vi "DIAdem Enqueue Request.vi"(7 "Queue Entry":enum16{"Front", "Back"}(ring), 8 "error in (no error)":errorcluster, 9 "timeout in ms (300000)":i32=300000, 10 "Wait for Completion? (f)":bool, 11 "DD_Report":T1) -> (0 "error out":errorcluster, 2 "timed out?":bool, 3 "Results":string)   [LabVIEW 2011]
uses:
  DIAdem Daemon Queue.ctl
  DIAdem Daemon Script Type.ctl
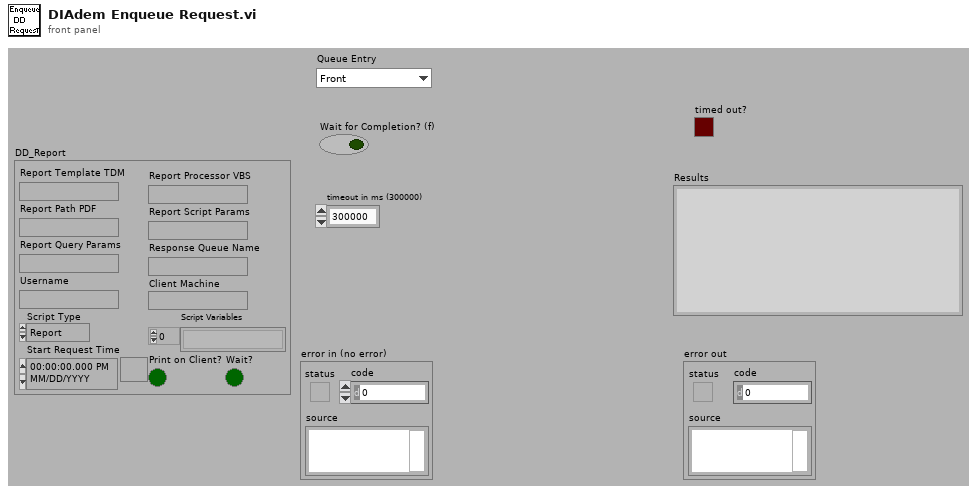
[diagram p1: front panel]
types:
  T1 = typedef "DIAdem Daemon Queue.ctl" = cluster{"Report Template TDM":path, "Report Processor VBS":path, "Report Path PDF":path, "Report Script Params":string, "Username":string, "Script Type":T2, "Report Query Params":string, "Client Machine":string, "Print on Client?":bool, "Response Queue Name":string, "Script Variables":string[], "Start Request Time":timestamp, "Wait?":bool}
  T2 = typedef "DIAdem Daemon Script Type.ctl" = enum16{"Report", "Query", "Script", "Datasheet", "Append", "Restart", "Stop"}
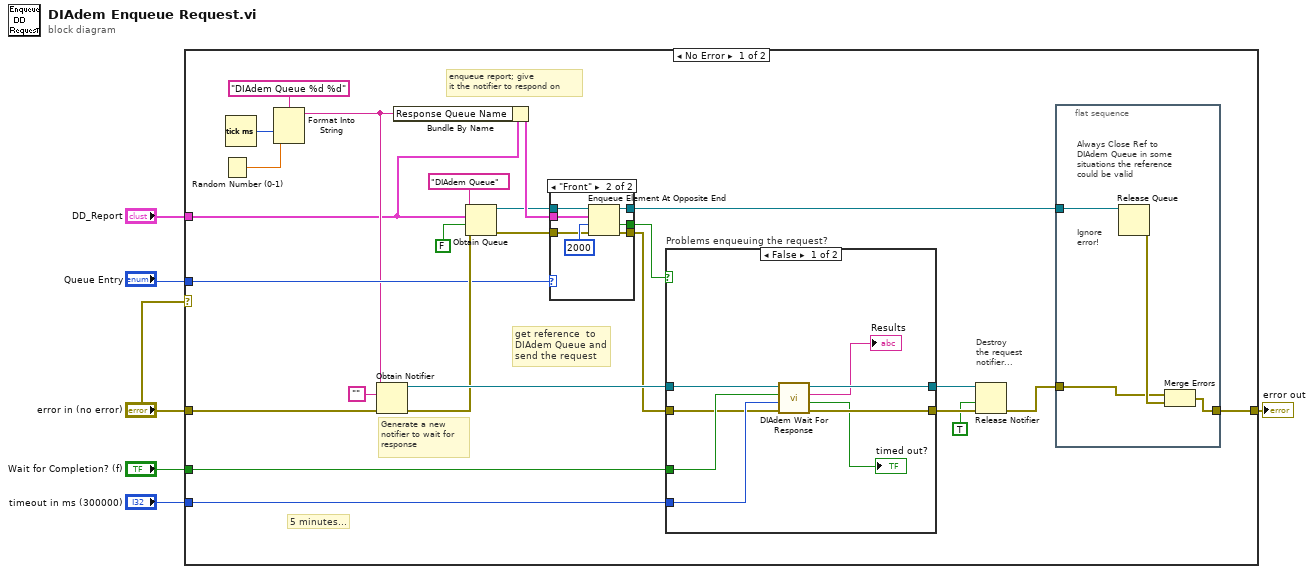
[diagram p0: block diagram]
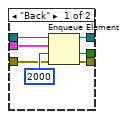
[diagram p2: hidden frame]
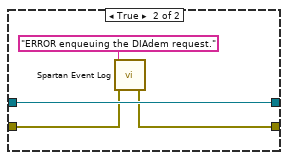
[diagram p3: hidden frame]
diagram:
  n1 = case shown="No Error" "error in (no error)" {
    tunnel: [w31 w62] -> w6
    tunnel: "error in (no error)" -> [w30 w62]
    tunnel: "DD_Report" -> [w10 _]
    tunnel: "Wait for Completion? (f)" -> [w26 _]
    tunnel: "timeout in ms (300000)" -> [w13 _]
    tunnel: "Queue Entry" -> [w12 _]
    frame No Error {
      # "Generate a new\nnotifier to wait for\nresponse"
      # "Destroy\nthe request\nnotifier..."
      # "5 minutes..."
      # "enqueue report; give\nit the notifier to respond on"
      # "get reference  to \nDIAdem Queue and\nsend the request"
      n2 = Random Number (0-1)() -> (number: 0 to 1=w7:dbl)
      n3 = Tick Count (ms)() -> (millisecond timer value=w8:u32)
      n4 = Format Into String(format string="DIAdem Queue %d %d" ("name (unnamed)"), w8, w7) -> (resulting string=w11:string)  [unwired: 2 in, 1 out]
      n5 = Obtain Notifier(name (unnamed)=w11, notification data type="", error in (no error)=w30) -> (notifier out=w29:refnum<notifier>, error out=w15:errorcluster)  [unwired: 1 in, 1 out]
      n6 = Bundle By Name(cluster=w10, "Response Queue Name"=w11) -> (w27:T1)
      n7 = Obtain Queue(name (unnamed)="DIAdem Queue", element data type=w10, create if not found? (T)=FALSE, error in (no error)=w15) -> (queue out=w22:refnum<queue>, error out=w23:errorcluster)  [unwired: 1 in, 1 out]
      n8 = case shown="\"Front\"" w12 {
        tunnel: w27 -> [w38 w45]
        tunnel: [w36 w43] -> w25
        tunnel: [w35 w42] -> w24
        tunnel: w23 -> [w34 w41]
        tunnel: w22 -> [w33 w40]
        tunnel: [w32 w39] -> w17
        frame "Back" {
          n9 = Enqueue Element(queue=w33, element=w38, timeout in ms (-1)=2000, error in (no error)=w34) -> (queue out=w32:refnum<queue>, timed out?=w35:bool, error out=w36:errorcluster)
        }
        frame "Front" {
          n10 = Enqueue Element At Opposite End(queue=w40, element=w45, timeout in ms (-1)=2000, error in (no error)=w41) -> (queue out=w39:refnum<queue>, timed out?=w42:bool, error out=w43:errorcluster)
        }
      }
      n11 = case "Problems enqueuing the request?" shown="False" w24 {
        tunnel: w25 -> [w54 w59]
        tunnel: w29 -> [w55 w61]
        tunnel: [w53 w58] -> w19
        tunnel: w26 -> [w56 _]
        tunnel: [w52 w61] -> w18
        tunnel: w13 -> [w57 _]
        frame False {
          n12 = call "DIAdem Wait For Response.vi"("error in (no error)"=w54, "timeout in ms (-1)"=w57, "Wait for Response? (f)"=w56, "notifier (NULL)"=w55) -> ("error out"=w53:errorcluster, "Timed Out?"=→"timed out?":bool, "Response"=→"Results":string, "dup notifier"=w52:refnum<notifier>)  [unwired: 4 out]
        }
        frame True {
          n13 = call "Spartan Event Log.vi"("error in (no error)"=w59, "message (\"\")"="ERROR enqueuing the DIAdem request." ("source")) -> ("error out"=w58:errorcluster)  [unwired: 6 in]
        }
      }
      n14 = Release Notifier(notifier=w18, force destroy? (F)=TRUE, error in (no error)=w19) -> (error out=w14:errorcluster)  [unwired: 2 out]
      n15 = flat-sequence {
        tunnel: w17 -> [w49]
        tunnel: w14 -> [w47]
        tunnel: [w46] -> w31
        frame #0 {
          # "Ignore\nerror!"
          # "Always Close Ref to \nDIAdem Queue in some\nsituations the reference\ncould be valid"
          n16 = Release Queue(queue=w49) -> (error out=w48:errorcluster)  [unwired: 1 in, 3 out]
          n17 = Merge Errors(w47, w48) -> (w46:errorcluster)
        }
      }
    }
    frame Error {
    }
  }
  "error out" <- w6
